vi "Configure Spectrum Emission Mask (Offset BandWidth).vi"(0 "VISA resource name":refnum<visa-resource-name>, 1 "SEM Resolution Bandwidth":i32[](array[ring]) items=["30 Hz", "100 Hz", "300 Hz", "1 kHz", "3 kHz", "10 kHz", "30 kHz", "100 kHz", "300 kHz", "1 MHz", "3 MHz", "50 kHz", "5 MHz", "10 MHz", "20 MHz"], 2 "SEM Auto Resolution Bandwidth":i32[](array[ring]) items=["Off", "On"], 5 "SEM Auto Video Bandwidth":i32[](array[ring]) items=["Off", "On"], 7 "SEM Video Bandwidth":i32[](array[ring]) items=["Off", "1 Hz", "3 Hz", "10 Hz", "30 Hz", "100 Hz", "300 Hz", "1 kHz", "3 kHz", "10 kHz", "30 kHz", "100 kHz", "300 kHz", "1 MHz", "3 MHz", "10 MHz", "5 kHz"], 9 "SEM Video Bandwidth Method":i32[](array[ring]) items=["Normal VBW", "Power VBW"], 11 "error in (no error)":errorcluster, 12 "SEM Auto Integrate Bandwidth":i32[](array[ring]) items=["Off", "On"], 13 "SEM Integrate Bandwidth":i32[](array[ring]) items=["30 Hz", "100 Hz", "300 Hz", "1 kHz", "3 kHz", "10 kHz", "30 kHz", "100 kHz", "300 kHz", "1 MHz", "3 MHz", "5 MHz", "10 MHz", "20 MHz"]) -> (4 "VISA resource name out":refnum<visa-resource-name>, 15 "error out":errorcluster)   [LabVIEW 2020, in "Anritsu Signal Analyzer Series.lvlib"]
doc: "Configures the setup for offset bandwidth of SEM measurement settings of the spectrum analyzer."
uses:
  Anritsu Signal Analyzer Series.lvlib
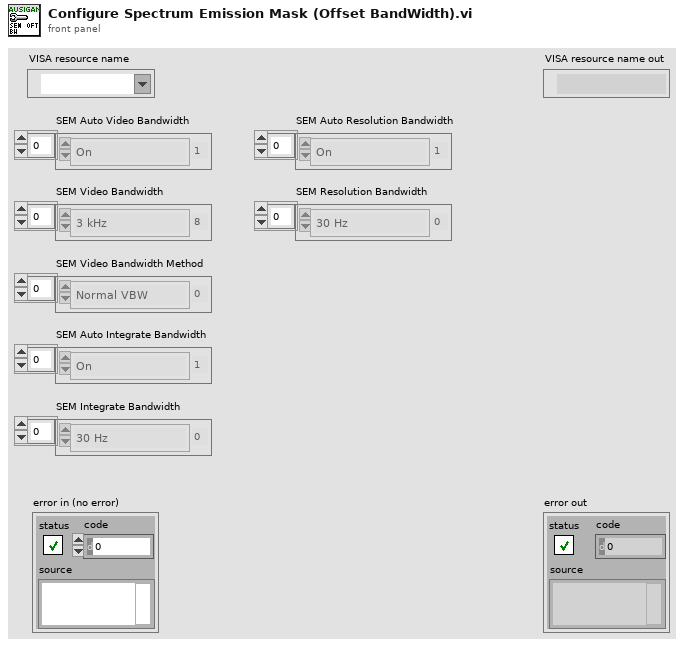
[diagram p1: front panel]
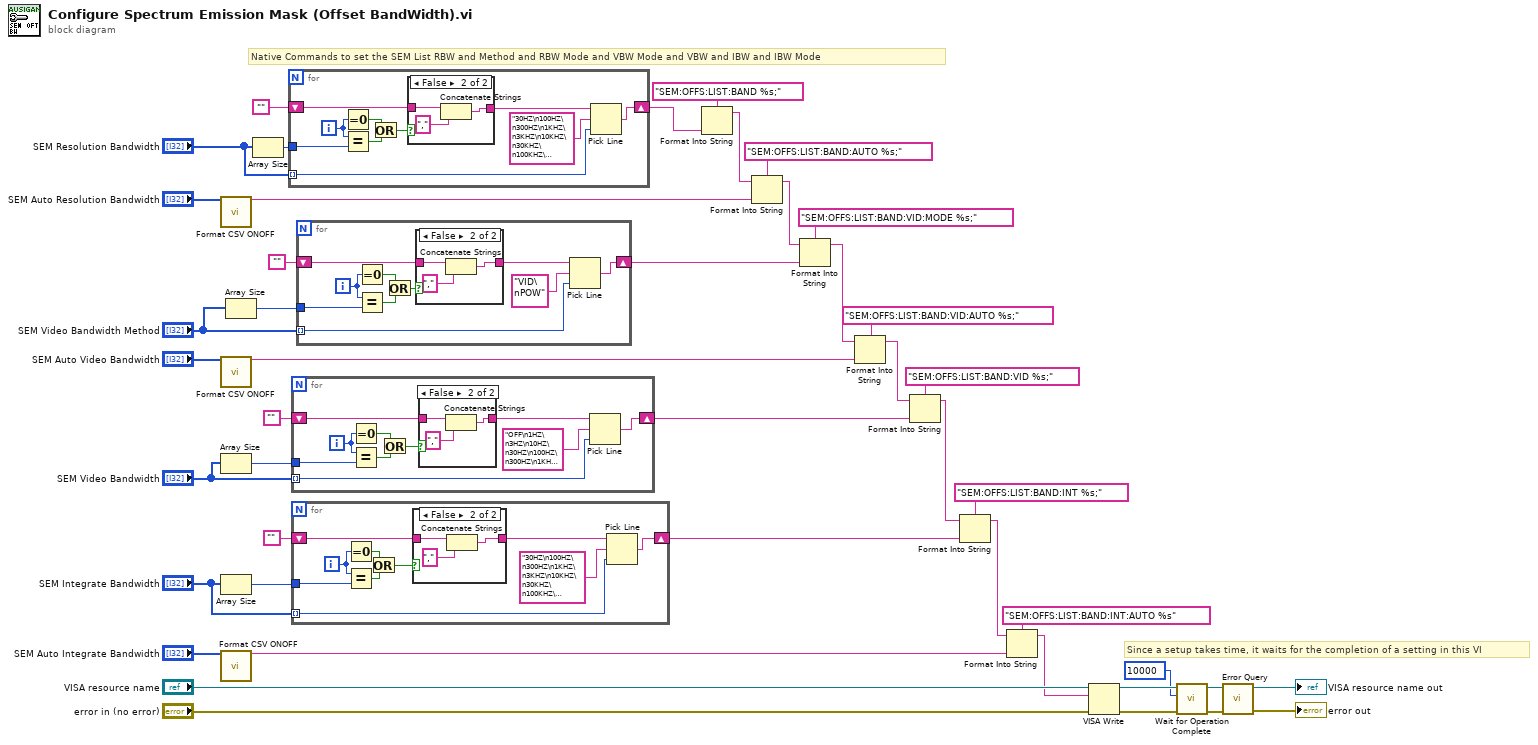
[diagram p0: block diagram]
diagram:
  # "Since a setup takes time, it waits for the completion of a setting in this VI"
  # "Native Commands to set the SEM List RBW and Method and RBW Mode and VBW Mode and VBW and IBW and IBW Mode"
  n1 = call "Format CSV ONOFF.vi"("Data_In"="SEM Auto Resolution Bandwidth") -> ("Data_out"=w26:string)  [unwired: 14 in]
  n2 = call "Format CSV ONOFF.vi"("Data_In"="SEM Auto Video Bandwidth") -> ("Data_out"=w25:string)  [unwired: 14 in]
  n3 = Array Size(array="SEM Video Bandwidth") -> (size(s)=w19:i32)
  n4 = Array Size(array="SEM Integrate Bandwidth") -> (size(s)=w17:i32)
  n5 = call "Format CSV ONOFF.vi"("Data_In"="SEM Auto Integrate Bandwidth") -> ("Data_out"=w24:string)  [unwired: 14 in]
  n6 = Array Size(array="SEM Video Bandwidth Method") -> (size(s)=w23:i32)
  n7 = Array Size(array="SEM Resolution Bandwidth") -> (size(s)=w27:i32)
  n8 = for {
    tunnel: "SEM Resolution Bandwidth" -> [w48] mode=indexing
    shift-right: [w46] -> w34
    shift-left: "" -> [w55]
    tunnel: w27 -> [w50]
    i -> [w51]
    n9 = Equal To 0?(x=w51) -> (x = 0?=w54:bool)
    n10 = Equal?(x=w51, y=w50) -> (x = y?=w53:bool)
    n11 = Or(x=w54, y=w53) -> (x .or. y?=w52:bool)
    n12 = case shown="False" w52 {
      tunnel: w55 -> [w56 w59]
      tunnel: [w56 w57] -> w47
      frame True {
      }
      frame False {
        n13 = Concatenate Strings(w59, "," ("string")) -> (w57:string)
      }
    }
    n14 = Pick Line(string ("")=w47, multi-line string="30HZ\n100HZ\n300HZ\n1KHZ\n3KHZ\n10KHZ\n30KHZ\n100KHZ\n300KHZ\n1MHZ\n3MHZ\n50KHZ\n5MHZ\n10MHZ\n20MHZ" ("複数行文字列"), line index=w48) -> (output string=w46:string)
  }
  n15 = for {
    tunnel: "SEM Video Bandwidth" -> [w61] mode=indexing
    shift-right: [w62] -> w18
    shift-left: "" -> [w69]
    tunnel: w19 -> [w64]
    i -> [w65]
    n16 = Equal To 0?(x=w65) -> (x = 0?=w68:bool)
    n17 = Equal?(x=w65, y=w64) -> (x = y?=w67:bool)
    n18 = Or(x=w68, y=w67) -> (x .or. y?=w66:bool)
    n19 = case shown="False" w66 {
      tunnel: w69 -> [w70 w73]
      tunnel: [w70 w71] -> w60
      frame True {
      }
      frame False {
        n20 = Concatenate Strings(w73, "," ("string")) -> (w71:string)
      }
    }
    n21 = Pick Line(string ("")=w60, multi-line string="OFF\n1HZ\n3HZ\n10HZ\n30HZ\n100HZ\n300HZ\n1KHZ\n3KHZ\n10KHZ\n30KHZ\n100KHZ\n300KHZ\n1MHZ\n3MHZ\n5MHZ\n10MHZ\n5KHZ" ("複数行文字列"), line index=w61) -> (output string=w62:string)
  }
  n22 = for {
    tunnel: "SEM Integrate Bandwidth" -> [w74] mode=indexing
    shift-right: [w75] -> w15
    shift-left: "" -> [w83]
    tunnel: w17 -> [w78]
    i -> [w79]
    n23 = Equal To 0?(x=w79) -> (x = 0?=w82:bool)
    n24 = Equal?(x=w79, y=w78) -> (x = y?=w81:bool)
    n25 = Or(x=w82, y=w81) -> (x .or. y?=w80:bool)
    n26 = case shown="False" w80 {
      tunnel: w83 -> [w84 w87]
      tunnel: [w84 w85] -> w76
      frame True {
      }
      frame False {
        n27 = Concatenate Strings(w87, "," ("string")) -> (w85:string)
      }
    }
    n28 = Pick Line(string ("")=w76, multi-line string="30HZ\n100HZ\n300HZ\n1KHZ\n3KHZ\n10KHZ\n30KHZ\n100KHZ\n300KHZ\n1MHZ\n3MHZ\n5MHZ\n10MHZ\n20MHZ" ("複数行文字列"), line index=w74) -> (output string=w75:string)
  }
  n29 = for {
    tunnel: "SEM Video Bandwidth Method" -> [w88] mode=indexing
    shift-right: [w89] -> w21
    shift-left: "" -> [w97]
    tunnel: w23 -> [w92]
    i -> [w93]
    n30 = Equal To 0?(x=w93) -> (x = 0?=w96:bool)
    n31 = Equal?(x=w93, y=w92) -> (x = y?=w95:bool)
    n32 = Or(x=w96, y=w95) -> (x .or. y?=w94:bool)
    n33 = case shown="False" w94 {
      tunnel: w97 -> [w98 w101]
      tunnel: [w98 w99] -> w90
      frame True {
      }
      frame False {
        n34 = Concatenate Strings(w101, "," ("string")) -> (w99:string)
      }
    }
    n35 = Pick Line(string ("")=w90, multi-line string="VID\nPOW" ("複数行文字列"), line index=w88) -> (output string=w89:string)
  }
  n36 = Format Into String(format string="SEM:OFFS:LIST:BAND %s;" ("_CommandSet"), w34) -> (resulting string=w6:string)  [unwired: 2 in, 1 out]
  n37 = Format Into String(format string="SEM:OFFS:LIST:BAND:AUTO %s;" ("_CommandSet"), initial string=w6, w26) -> (resulting string=w12:string)  [unwired: 1 in, 1 out]
  n38 = Format Into String(format string="SEM:OFFS:LIST:BAND:VID:MODE %s;" ("_CommandSet"), initial string=w12, w21) -> (resulting string=w13:string)  [unwired: 1 in, 1 out]
  n39 = Format Into String(format string="SEM:OFFS:LIST:BAND:VID:AUTO %s;" ("_CommandSet"), initial string=w13, w25) -> (resulting string=w14:string)  [unwired: 1 in, 1 out]
  n40 = Format Into String(format string="SEM:OFFS:LIST:BAND:VID %s;" ("_CommandSet"), initial string=w14, w18) -> (resulting string=w11:string)  [unwired: 1 in, 1 out]
  n41 = Format Into String(format string="SEM:OFFS:LIST:BAND:INT %s;" ("_CommandSet"), initial string=w11, w15) -> (resulting string=w10:string)  [unwired: 1 in, 1 out]
  n42 = Format Into String(format string="SEM:OFFS:LIST:BAND:INT:AUTO %s" ("_CommandSet"), initial string=w10, w24) -> (resulting string=w9:string)  [unwired: 1 in, 1 out]
  n43 = VISA Write(VISA resource name="VISA resource name", write buffer=w9, error in (no error)="error in (no error)") -> (VISA resource name out=w5:refnum<visa-resource-name>, error out=w4:errorcluster)  [unwired: 1 out]
  n44 = call "Wait for Operation Complete.vi"("error in (no error)"=w4, "Maximum Time (10000mSec)"=10000, "VISA resource name"=w5) -> ("error out"=w8:errorcluster, "VISA resource name out"=w7:refnum<visa-resource-name>)  [unwired: 7 in]
  n45 = call "Error Query.vi"("error in (no error)"=w8, "VISA resource name"=w7) -> ("error out"=→"error out":errorcluster, "VISA resource name out"=→"VISA resource name out":refnum<visa-resource-name>)  [unwired: 6 in, 2 out]
